vi "Actor Create.vi"(9 "Nest Alias":string, 10 "Nest Actor":refnum<class "Actor.lvclass">, 11 "Dev Actor in":refnum<class "Dev Actor.lvclass">) -> (0 "error out":errorcluster, 3 "Dev Actor out":refnum<class "Dev Actor.lvclass">)   [LabVIEW 2021, in "Dev Actor.lvlib" / "Dev Actor.lvclass"]
uses:
  Dev Actor.lvclass
  LVCAM/LVCAM/Actor/Actor.lvclass
  Dev Actor.lvclass/Dev Actor.ctl
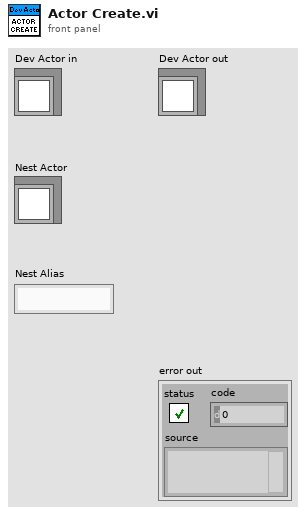
[diagram p1: front panel]
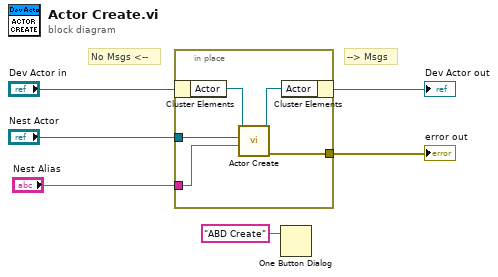
[diagram p0: block diagram]
diagram:
  # "--> Msgs"
  # "No Msgs <--"
  n1 = in-place {
    in-place-border: "Nest Actor" -> [w9]
    in-place-border: "Nest Alias" -> [w7]
    in-place-border: [w8] -> w2
    n2 = in-place-cluster #1("Dev Actor in") -> ("Actor"=w11:refnum<class "Actor.lvclass">)
    n3 = call-dynamic "Actor Create.vi"("Nest Alias"=w7, "Nest Actor"=w9, "Actor Create in"=w11) -> ("error out"=w8:errorcluster, "Actor Create out"=w10:refnum<class "Actor.lvclass">)  [unwired: 7 in]
    n4 = in-place-cluster #1("Actor"=w10) -> (→"Dev Actor out":refnum<class "Dev Actor.lvclass">)
  }
  "error out" <- w2
  n5 = One Button Dialog(message="ABD Create") -> ()  [unwired: 1 in, 1 out]
